vi "remove class zeros.vi"(7 "Array In":dbl[][](array[numeric])) -> (3 "Array Out":dbl[][](array[numeric]))   [LabVIEW 2012]
panel:
  # "// Andrew Combs\n// 02-23-13\n// Searches a 2D array and removes any row with a zero in Col 8\n// Input:     2D array of goals in standard format LANDSCAPE\n// Output:  2D array of goals in standard format LANDSCAPE minus all class zero targets"
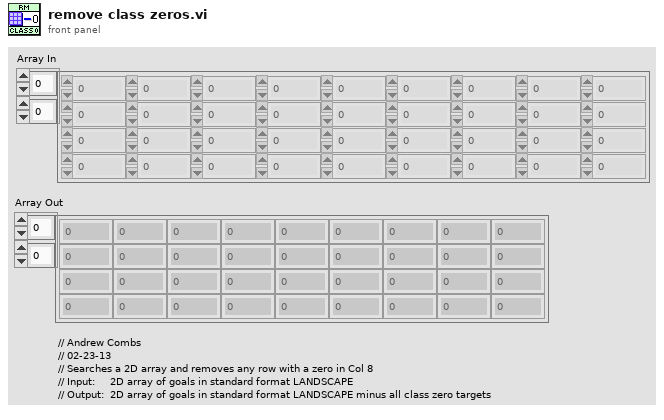
[diagram p1: front panel]
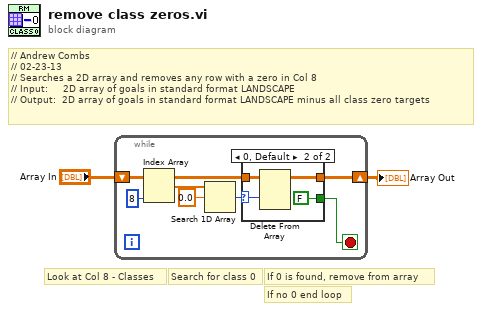
[diagram p0: block diagram]
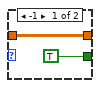
[diagram p2: hidden frame]
diagram:
  # "// Andrew Combs\n// 02-23-13\n// Searches a 2D array and removes any row with a zero in Col 8\n// Input:     2D array of goals in standard format LANDSCAPE\n// Output:  2D array of goals in standard format LANDSCAPE minus all class zero targets"
  # "If no 0 end loop"
  # "If 0 is found, remove from array"
  # "Search for class 0"
  # "Look at Col 8 - Classes"
  n1 = while {
    shift-right: [w3] -> w1
    shift-left: "Array In" -> [w6]
    stop <- w4 stop-if-true
    n2 = Index Array(array=w6, index (col)=8 ("index (row)")) -> (element=w9:dbl[])  [unwired: 1 in]
    n3 = Search 1D Array(1D array=w9, element=0.0) -> (index of element=w7:i32)  [unwired: 1 in]
    n4 = case shown="0, Default" w7 {
      selector: w7 -> [_ w13]
      tunnel: w6 -> [w11 w15]
      tunnel: [w11 w14] -> w3
      tunnel: [TRUE FALSE] -> w4
      frame -1 {
      }
      frame 0, Default {
        n5 = Delete From Array(array=w15, index (row)=w13) -> (array with subset deleted=w14:dbl[][])  [unwired: 2 in, 1 out]
      }
    }
  }
  "Array Out" <- w1
